vi "Less Than.vi"(10 "Numeric 3":dbl, 11 "Numeric in":dbl) -> (3 "Numeric out":dbl)   [LabVIEW 2016]
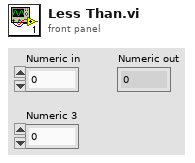
[diagram p1: front panel]
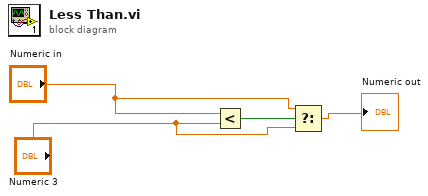
[diagram p0: block diagram]
diagram:
  n1 = Less?(x="Numeric in", y="Numeric 3") -> (x < y?=w1:bool)
  n2 = Select(t="Numeric in", s=w1, f="Numeric 3") -> (s? t:f=→"Numeric out":dbl)
